vi "afonin_et7026(1).vi"() -> ()   [LabVIEW 2012]
panel:
  in  "Path":path
  out "Торр":dbl format="%#_2g"
  out "Па":dbl format="%#_2e"
  out "мбар":dbl format="%#_2g"
  out "Торр":dbl(graph)
  out "Waveform Chart":dbl(graph)
  in  "Remote Port":u16=502
  in  "Remote IP for 7026":string="127.0.0.1"
  in  "Stop":bool
  out "AI":u16[](array[numeric])
  out "DI":bool[](array[boolean]) caption="Slave Discrete Inputs"
  in  "DO":bool[](array[boolean])=[FALSE, FALSE, FALSE, FALSE] caption="Coils to Write"
  in  "AO":u16[](array[numeric])=[0, 0, 0, 0] caption="Registers to Write"
  # "192.168.0.122"
  # "Data to write to the slave"
  # "Slave Read-only Registers"
  # "DO 0"
  # "DO 1"
  # "DI 0"
  # "DI 1"
  # "AO 0"
  # "AO 1"
  # "AI 0"
  # "AI 1"
  # "AI 2"
  # "AI 3"
  # "AI 4"
  # "AI 5"
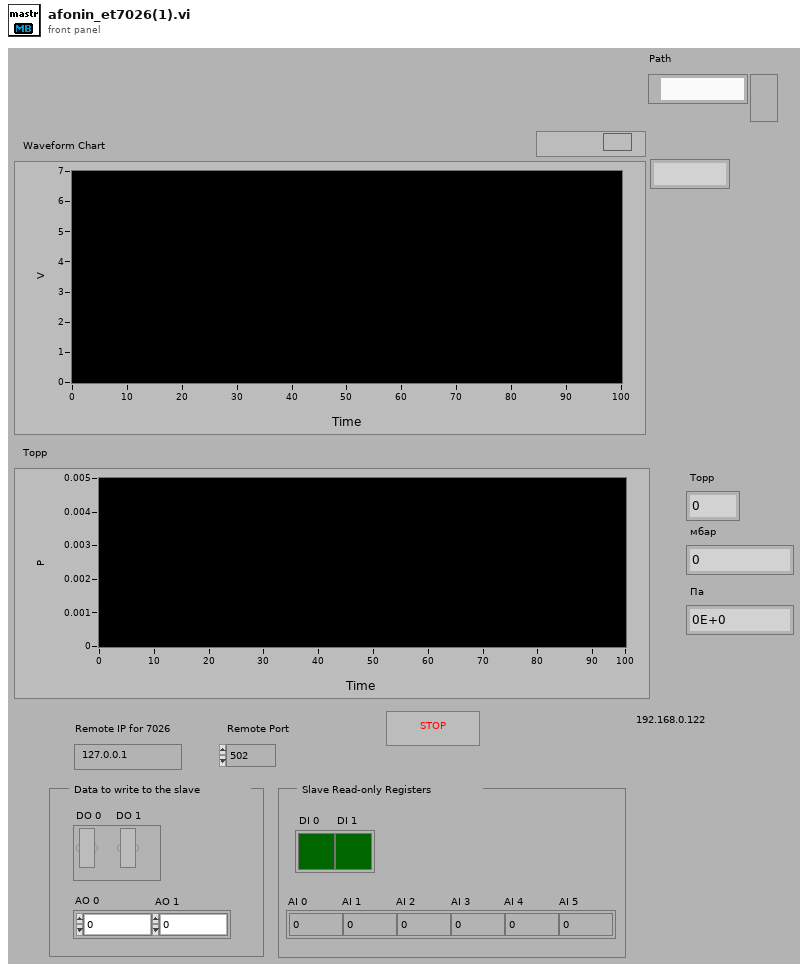
[diagram p1: front panel]
types:
  T1 = typedef "MB Modbus Command.ctl" = cluster{"Function Code":u8, "Starting Address":u16, "Quantity":u16, "Data":u16[], "Discrete":bool[]}
  T2 = enum16{"replace", "open", "create", "open or create", "replace or create", "replace or create with confirmation"}
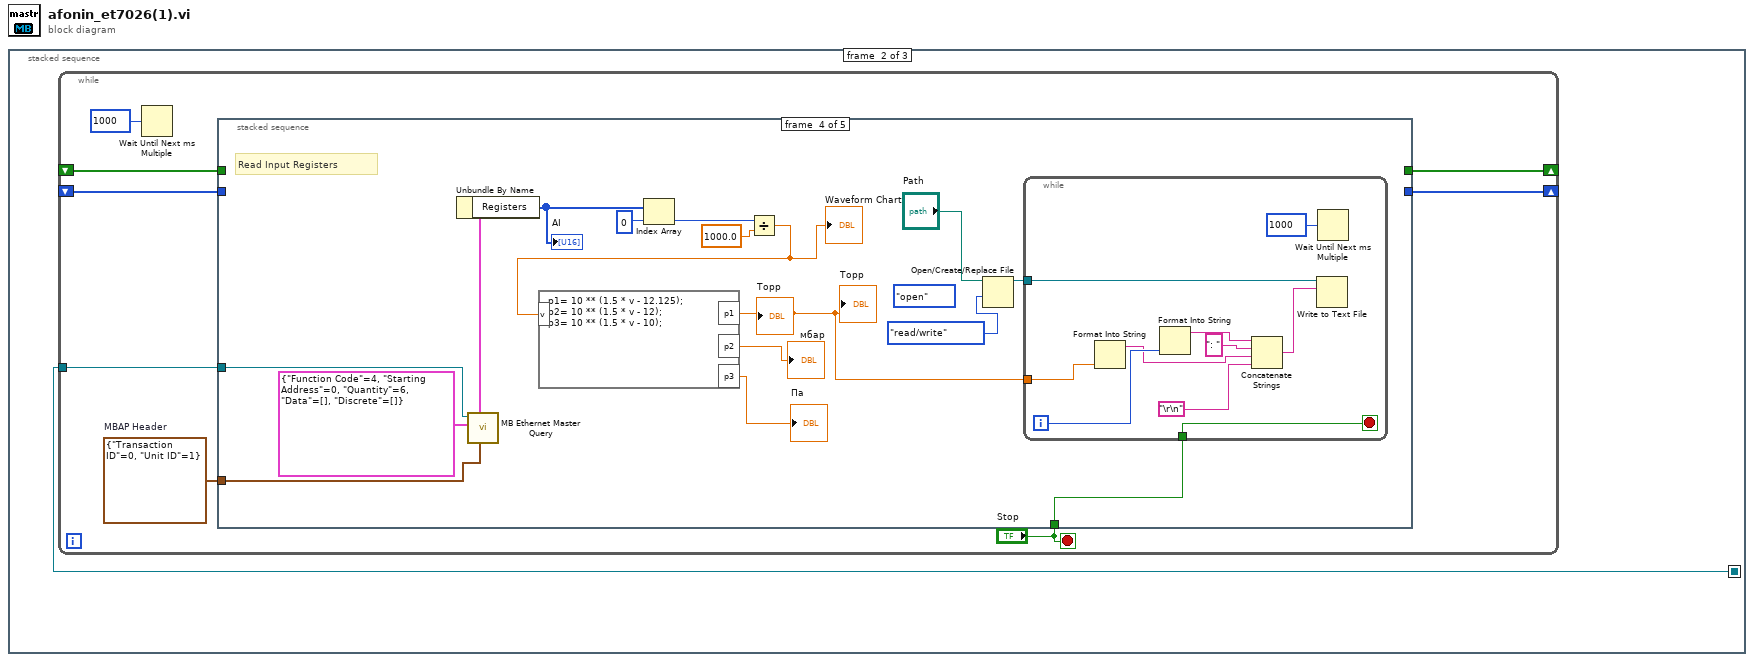
[diagram p0: block diagram]
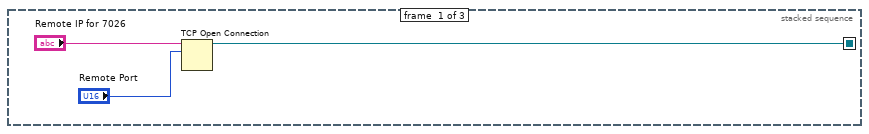
[diagram p2: hidden frame]
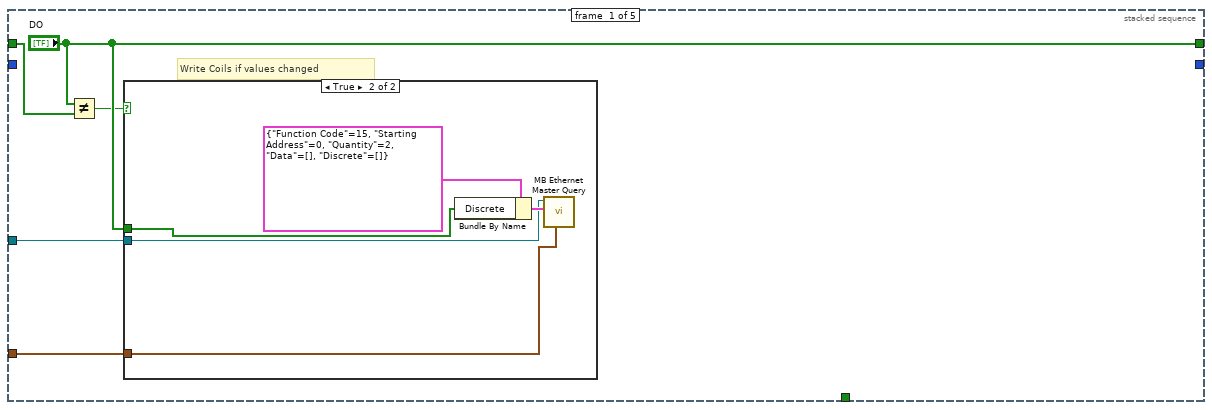
[diagram p3: hidden frame]
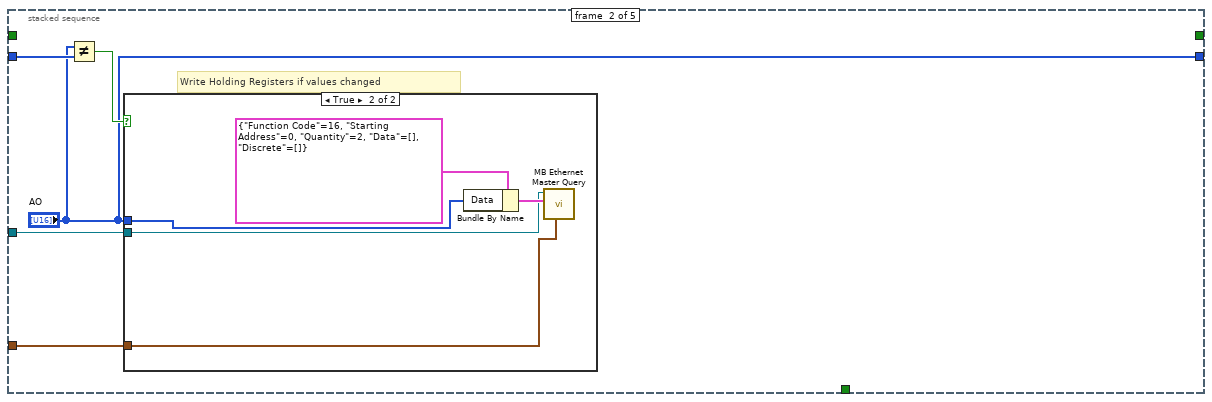
[diagram p5: hidden frame]
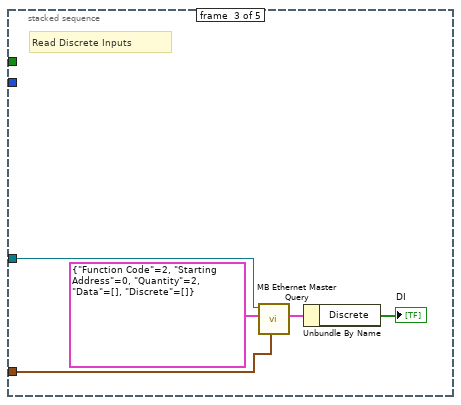
[diagram p7: hidden frame]
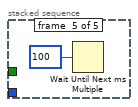
[diagram p8: hidden frame]
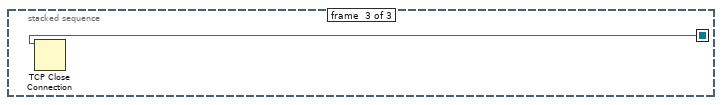
[diagram p9: hidden frame]
diagram:
  n1 = stacked-sequence {
    seq-local: [w1 _ _] -> [_ w4 w65]
    frame #0 {
      n2 = TCP Open Connection(address="Remote IP for 7026", remote port or service name="Remote Port") -> (connection ID=w1:refnum<k5>)  [unwired: 3 in, 1 out]
    }
    frame #1 {
      n3 = while {
        tunnel: w4 -> [w12]
        shift-right: [w10] -> _
        shift-left: _ -> [w11]
        shift-right: [w8] -> _
        shift-left: _ -> [w9]
        stop <- "Stop" stop-if-true
        w6 = cluster{"Transaction ID":u16, "Unit ID":u8} {"Transaction ID"=0, "Unit ID"=1}  # MBAP Header
        n4 = Wait Until Next ms Multiple(millisecond multiple=u32 1000) -> ()  [unwired: 1 out]
        n5 = stacked-sequence {
          tunnel: w12 -> [w17 w27 w37 w53 _]
          tunnel: w11 -> [w16 _ _ _ _]
          tunnel: ["DO" _ _ _ _] -> w10
          tunnel: w9 -> [_ w25 _ _ _]
          tunnel: [_ "AO" _ _ _] -> w8
          tunnel: w6 -> [w13 w23 w33 w50 _]
          tunnel: "Stop" -> [_ _ _ w38 _]
          frame #0 {
            # "Write Coils if values changed"
            n6 = Not Equal?(x="DO", y=w16) -> (x != y?=w14:bool)
            n7 = case shown="True" w14 {
              tunnel: w17 -> [_ w20]
              tunnel: "DO" -> [_ w19]
              tunnel: w13 -> [_ w18]
              frame False {
              }
              frame True {
                n8 = Bundle By Name(cluster=T1 {"Function Code"=15, "Starting Address"=0, "Quantity"=2, "Data"=[], "Discrete"=[]} ("MODBUS Command"), "Discrete"=w19) -> (w21:T1)
                n9 = call "MB Ethernet Master Query.vi"("MBAP Header"=w18, "Modbus Command"=w21, "TCP Connection Refnum in"=w20) -> ()  [unwired: 4 in, 5 out]
              }
            }
          }
          frame #1 {
            # "Write Holding Registers if values changed"
            n10 = Not Equal?(x="AO", y=w25) -> (x != y?=w26:bool)
            n11 = case shown="True" w26 {
              tunnel: w27 -> [_ w30]
              tunnel: "AO" -> [_ w29]
              tunnel: w23 -> [_ w28]
              frame False {
              }
              frame True {
                n12 = Bundle By Name(cluster=T1 {"Function Code"=16, "Starting Address"=0, "Quantity"=2, "Data"=[], "Discrete"=[]} ("MODBUS Command"), "Data"=w29) -> (w31:T1)
                n13 = call "MB Ethernet Master Query.vi"("MBAP Header"=w28, "Modbus Command"=w31, "TCP Connection Refnum in"=w30) -> ()  [unwired: 4 in, 5 out]
              }
            }
          }
          frame #2 {
            # "Read Discrete Inputs"
            n14 = call "MB Ethernet Master Query.vi"("MBAP Header"=w33, "Modbus Command"=T1 {"Function Code"=2, "Starting Address"=0, "Quantity"=2, "Data"=[], "Discrete"=[]} ("MODBUS Command"), "TCP Connection Refnum in"=w37) -> ("Registers"=w36:cluster{"Registers":u16[], "Discrete":bool[]})  [unwired: 4 in, 4 out]
            n15 = Unbundle By Name(w36) -> ("Discrete"=→"DI":bool[])
          }
          frame #3 {
            (unwired) T2."open"
            # "Read Input Registers"
            n16 = call "MB Ethernet Master Query.vi"("MBAP Header"=w50, "Modbus Command"=T1 {"Function Code"=4, "Starting Address"=0, "Quantity"=6, "Data"=[], "Discrete"=[]} ("MODBUS Command"), "TCP Connection Refnum in"=w53) -> ("Registers"=w52:cluster{"Registers":u16[], "Discrete":bool[]})  [unwired: 4 in, 4 out]
            n17 = Unbundle By Name(w52) -> ("Registers"=w49:u16[])
            "AI" <- w49
            n18 = Index Array(array=w49, index=0) -> (element=w46:u16)
            n19 = Divide(x=w46, y=1000.0) -> (x/y=w45:dbl)
            "Waveform Chart" <- w45
            n20 = formula code="p1= 10 ** (1.5 * v - 12.125);\np2= 10 ** (1.5 * v - 12);\np3= 10 ** (1.5 * v - 10);"("v"=w45) -> ("p1"=w39:dbl, "p2"=→"мбар":dbl, "p3"=→"Па":dbl)
            "Торр" <- w39
            "Торр" <- w39
            n21 = Open/Create/Replace File(file path (use dialog)="Path", access (0:read/write)=enum16{"read/write", "read-only", "write-only"}."read/write") -> (refnum out=w40:refnum<file>)  [unwired: 4 in, 2 out]
            n22 = while {
              tunnel: w40 -> [w63]
              tunnel: w39 -> [w62]
              tunnel: w38 -> [w54]
              i -> [w61]
              stop <- w54 stop-if-true
              n23 = Format Into String(w62) -> (resulting string=w58:string)  [unwired: 3 in, 1 out]
              n24 = Format Into String(w61) -> (resulting string=w60:string)  [unwired: 3 in, 1 out]
              n25 = Concatenate Strings(w60, ": " ("string"), w58, "\r\n") -> (w57:string)
              n26 = Write to Text File(file (use dialog)=w63, text=w57) -> ()  [unwired: 2 in, 3 out]
              n27 = Wait Until Next ms Multiple(millisecond multiple=u32 1000) -> ()  [unwired: 1 out]
            }
          }
          frame #4 {
            n28 = Wait Until Next ms Multiple(millisecond multiple=u32 100) -> ()  [unwired: 1 out]
          }
        }
      }
    }
    frame #2 {
      n29 = TCP Close Connection(connection ID=w65) -> ()  [unwired: 2 in, 2 out]
    }
  }
